vi "playNote.vi"(1 "B":bool, 2 "A":bool, 3 "G":bool, 4 "F":bool, 5 "E":bool, 6 "D":bool, 7 "C":bool) -> (0 "freq":dbl)   [LabVIEW 2014]
uses:
  <vilib>/imath/engines/lvmath2/RunTimeEngine/Managers/WorkSpace/UID Generator.vi
  <vilib>/imath/engines/lvmath2/RunTimeEngine/RunTimeType/NIMS_RunTimeType_From StrictType (excl LVString).vi
  <instcachedir>/0/NIMS_RunTimeType_From StrictType (excl LVString)_15A5391EEA9C4AACB9955AC755B83D29.lvgen/NIMS_RunTimeType_From StrictType (excl LVString)_15A5391EEA9C4AACB9955AC755B83D29_000.vi
  <vilib>/imath/engines/lvmath2/RunTimeEngine/LocalVariableDefStatement/MC_LocalVariableDefStatement_Display.vi
  <vilib>/imath/engines/lvmath2/RunTimeEngine/Managers/SymbolTable/Clear UID.vi
  <vilib>/imath/engines/lvmath2/RunTimeEngine/NodeEndStatement/NIMS_NodeEndStatement_Output.vi
  <instcachedir>/0/NIMS_NodeEndStatement_Output_53EC0D466D134D7ABD903AC30B43404B.lvgen/NIMS_NodeEndStatement_Output_53EC0D466D134D7ABD903AC30B43404B_001.vi
  <vilib>/imath/engines/lvmath2/RunTimeEngine/ErrorHandling/NIMS_Finalize Error.vi
  <vilib>/imath/engines/lvmath2/RunTimeEngine/Managers/SymbolTable/NIMS_WorkSpace.lvlib
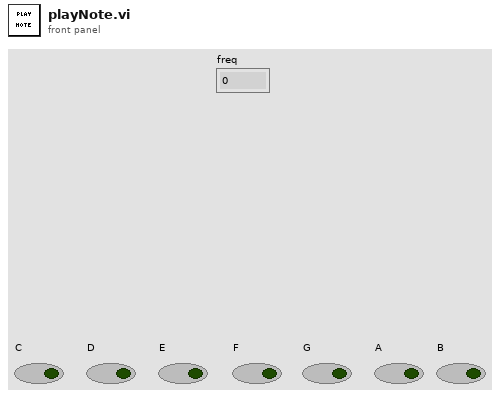
[diagram p1: front panel]
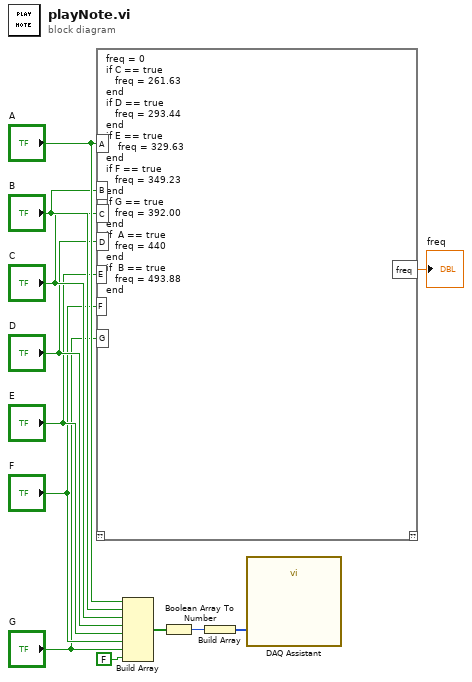
[diagram p0: block diagram]
diagram:
  n1 = mathscript code="freq = 0\nif C == true\n   freq = 261.63\nend\nif D == true\n   freq = 293.44\nend\nif E == true\n    freq = 329.63\nend\nif F == true\n   freq = 349.23\nend\nif G == true \n   freq = 392.00\nend\nif  A == true\n   freq = 440\nend\nif  B == true\n   freq = 493.88\nend"("A"="A", "B"="B", "C"="C", "D"="D", "E"="E", "F"="F", "G"="G") -> ("freq"=→"freq":dbl)  [unwired: 1 in, 1 out]
  n2 = Build Array("A", "B", "C", "D", "E", "F", "G", FALSE) -> (w9:bool[])
  n3 = Boolean Array To Number(Boolean array=w9) -> (number=w12:u32)
  n4 = Build Array(w12) -> (w11:u32[])
  n5 = call "DAQ Assistant"("data"=w11) -> ()  [unwired: 17 in, 2 out]
